vi "Launch New Chat Window.vi"(8 "error in (no error)":errorcluster, 11 "Server in":refnum<class "Server.lvclass">) -> (0 "error out":errorcluster, 3 "Server out":refnum<class "Server.lvclass">)   [LabVIEW 2015, in "Server.lvlib" / "Server.lvclass"]
uses:
  Server.lvclass
  Chat Window Model/Chat Window Model/Chat Window Model.lvclass
  Server Messages/Status Update Msg/Status Update Msg.lvclass
  Server Messages/Direct Message Recieved Msg/Direct Message Recieved Msg.lvclass
  Server Messages/New Reference Recieved Msg/New Reference Recieved Msg.lvclass
  Chat Window Model/Chat Window Model/Chat Window Model.lvclass/Chat Window Model.ctl
  <vilib>/ActorFramework/Actor/Actor.lvclass/Actor.ctl
  <vilib>/ActorFramework/Message Enqueuer/Message Enqueuer.lvclass/Message Enqueuer.ctl
  Server.lvclass/Server.ctl
  Server Messages/Enable Controls Msg/Enable Controls Msg.lvclass/Enable Controls Msg.ctl
  Chat Window Model/Chat Window Model Messages/Update Status Log Msg/Update Status Log Msg.lvclass/Update Status Log Msg.ctl
  Chat Window Model/Chat Window Model Messages/Update Online List Msg/Update Online List Msg.lvclass/Update Online List Msg.ctl
  <vilib>/ActorFramework/Message Enqueuer/Init from Existing Queue.vi
  <vilib>/ActorFramework/Message Enqueuer/Enqueue.vi
  <vilib>/ActorFramework/Message Priority Queue/Priority Enqueue.vi
  <vilib>/ActorFramework/Message Enqueuer/Message Enqueuer.lvclass
  Server Messages/Enable Controls Msg/Enable Controls Msg.lvclass
  Chat Window Model/Chat Window Model Messages/Update Status Log Msg/Update Status Log Msg.lvclass
  Chat Window Model/Chat Window Model Messages/Update Online List Msg/Update Online List Msg.lvclass
  <vilib>/ActorFramework/Actor/Actor.lvclass
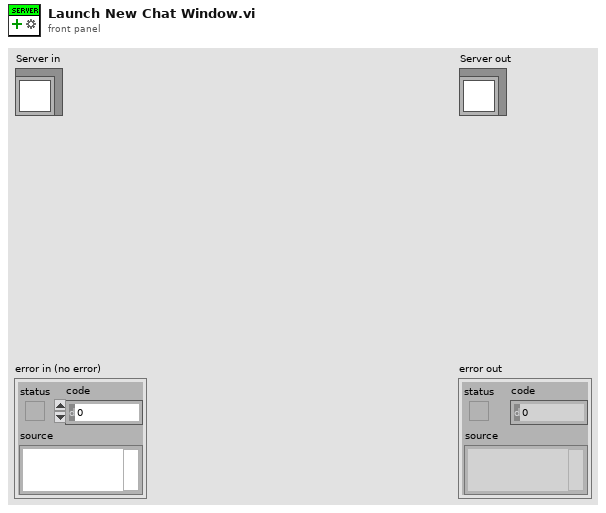
[diagram p1: front panel]
types:
  T1 = enum8{"Enabled", "Disabled", "Disabled and Grayed Out"}
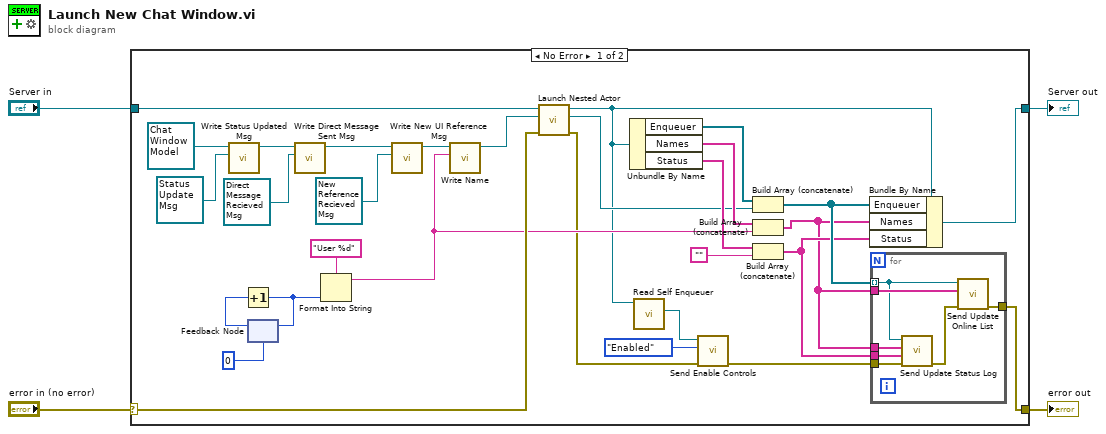
[diagram p0: block diagram]
diagram:
  n1 = case shown="No Error" "error in (no error)" {
    selector: "error in (no error)" -> [w33 w43]
    tunnel: [w13 w43] -> w3
    tunnel: [w17 w42] -> w1
    tunnel: "Server in" -> [w34 w42]
    frame No Error {
      n2 = call "Write Status Updated Msg.vi"("Chat Window Model.lvlib:Status Updated Msg.lvclass"=refnum<class "Status Update Msg.lvclass"> refnum ("Server.lvlib:Status Update Msg.lvclass"), "Chat Window Model in"=refnum<class "Chat Window Model.lvclass"> refnum ("Chat Window Model.lvlib:Chat Window Model.lvclass")) -> ("Chat Window Model out"=w25:refnum<class "Chat Window Model.lvclass">)  [unwired: 9 in]
      n3 = feedback #1(0) -> (w30:i32)
      n4 = Increment(x=w30) -> (x+1=w28:i32)
      n5 = feedback-in #1(w28) -> ()
      n6 = call "Write Direct Message Sent Msg.vi"("Chat Window Model.lvlib:Direct Message Sent Msg.lvclass"=refnum<class "Direct Message Recieved Msg.lvclass"> refnum ("Server.lvlib:Direct Message Recieved Msg.lvclass"), "Chat Window Model in"=w25) -> ("Chat Window Model out"=w7:refnum<class "Chat Window Model.lvclass">)  [unwired: 9 in]
      n7 = Format Into String(format string="User %d", w28) -> (resulting string=w19:string)  [unwired: 2 in, 1 out]
      n8 = call "Write New UI Reference Msg.vi"("Chat Window Model.lvlib:New UI Reference Msg.lvclass"=refnum<class "New Reference Recieved Msg.lvclass"> refnum ("Server.lvlib:New Reference Recieved Msg.lvclass"), "Chat Window Model in"=w7) -> ("Chat Window Model out"=w6:refnum<class "Chat Window Model.lvclass">)  [unwired: 9 in]
      n9 = call "Write Name.vi"("Name"=w19, "Chat Window Model in"=w6) -> ("Chat Window Model out"=w32:refnum<class "Chat Window Model.lvclass">)  [unwired: 8 in, 1 out]
      n10 = call <vilib>:"Launch Nested Actor.vi"("error in (no error)"=w33, "Nested Actor"=w32, "Caller Actor in"=w34) -> ("error out"=w11:errorcluster, "Nested Actor's Enqueuer"=w20:refnum<class "Message Enqueuer.lvclass">, "Caller Actor out"=w10:refnum<class "Server.lvclass">)  [unwired: 6 in]
      n11 = Unbundle By Name(w10) -> ("Enqueuer"=w23:refnum<class "Message Enqueuer.lvclass">[], "Names"=w22:string[], "Status"=w21:string[])
      n12 = call <vilib>:"Read Self Enqueuer.vi"("Actor"=w10) -> ("Self Enqueuer"=w9:refnum<class "Message Enqueuer.lvclass">)  [unwired: 10 in]
      n13 = call "Send Enable Controls.vi"("error in (no error)"=w11, "Disabled"=T1."Enabled", "Message Enqueuer"=w9) -> ("error out"=w12:errorcluster)  [unwired: 7 in, 1 out]
      n14 = Build Array (concatenate)(w23, w20) -> (w16:refnum<class "Message Enqueuer.lvclass">[])
      n15 = Build Array (concatenate)(w22, w19) -> (w14:string[])
      n16 = Build Array (concatenate)(w21, "") -> (w15:string[])
      n17 = Bundle By Name(cluster=w10, "Enqueuer"=w16, "Names"=w14, "Status"=w15) -> (w17:refnum<class "Server.lvclass">)
      n18 = for {
        tunnel: w16 -> [w40] mode=indexing
        tunnel: w14 -> [w41]
        tunnel: w15 -> [w39]
        tunnel: w14 -> [w38]
        tunnel: [w36] -> w13
        tunnel: w12 -> [w35]
        n19 = call "Send Update Status Log.vi"("error in (no error)"=w35, "Status List"=w39, "Names"=w38, "Message Enqueuer"=w40) -> ("error out"=w37:errorcluster)  [unwired: 6 in, 1 out]
        n20 = call "Send Update Online List.vi"("error in (no error)"=w37, "Online Users"=w41, "Message Enqueuer"=w40) -> ("error out"=w36:errorcluster)  [unwired: 7 in, 1 out]
      }
    }
    frame Error {
    }
  }
  "error out" <- w3
  "Server out" <- w1
